vi "translate_commands.vi"(11 "data":dbl[](array[numeric])) -> (0 "Numeric":dbl, 1 "Boolean 3":bool, 2 "Waveform":dbl, 3 "Boolean 4":bool, 4 "Boolean 2":bool, 5 "Boolean":bool, 6 "Boolean 5":bool)   [LabVIEW 2019]
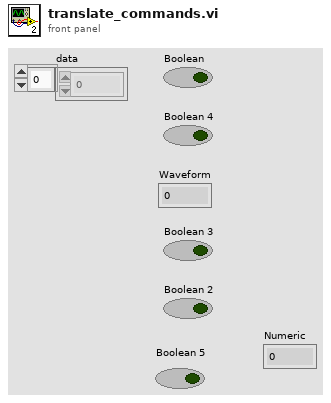
[diagram p1: front panel]
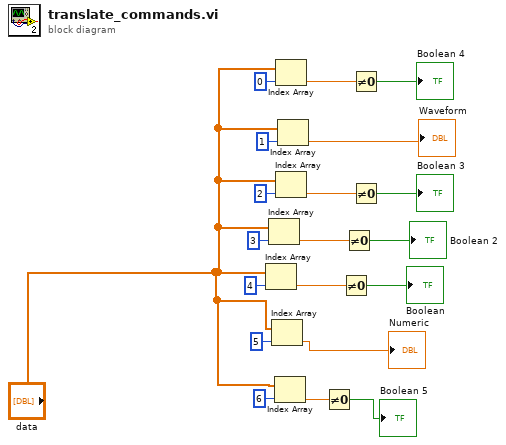
[diagram p0: block diagram]
diagram:
  n1 = Index Array(array="data", index=4) -> (element=w17:dbl)
  n2 = Index Array(array="data", index=3) -> (element=w14:dbl)
  n3 = Index Array(array="data", index=5) -> (element=→"Numeric":dbl)
  n4 = Index Array(array="data", index=6) -> (element=w2:dbl)
  n5 = Index Array(array="data", index=0) -> (element=w8:dbl)
  n6 = Index Array(array="data", index=2) -> (element=w11:dbl)
  n7 = Index Array(array="data", index=1) -> (element=→"Waveform":dbl)
  n8 = Not Equal To 0?(x=w2) -> (x != 0?=→"Boolean 5":bool)
  n9 = Not Equal To 0?(x=w17) -> (x != 0?=→"Boolean":bool)
  n10 = Not Equal To 0?(x=w14) -> (x != 0?=→"Boolean 2":bool)
  n11 = Not Equal To 0?(x=w8) -> (x != 0?=→"Boolean 4":bool)
  n12 = Not Equal To 0?(x=w11) -> (x != 0?=→"Boolean 3":bool)
